vi "Random Competition.vi"() -> ()   [LabVIEW 2025]
uses:
  <vilib>/numeric/Random Number (Range) DBL.vi
panel:
  out "Iteration Count":i32
  out "Winner B":bool
  out "Tie":bool
  out "Winner A":bool
  out "Points B":dbl
  out "Points A":dbl
  out "Random Number B":dbl
  out "Random Number A":dbl
  in  "Number of Iterations":i32 min=0 step=1
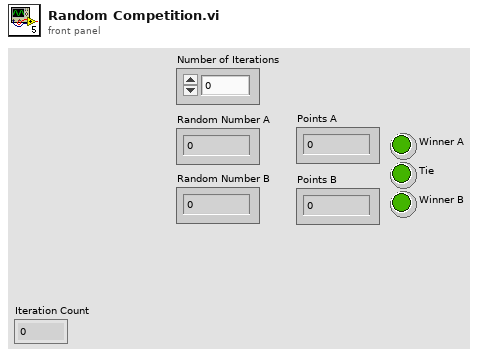
[diagram p1: front panel]
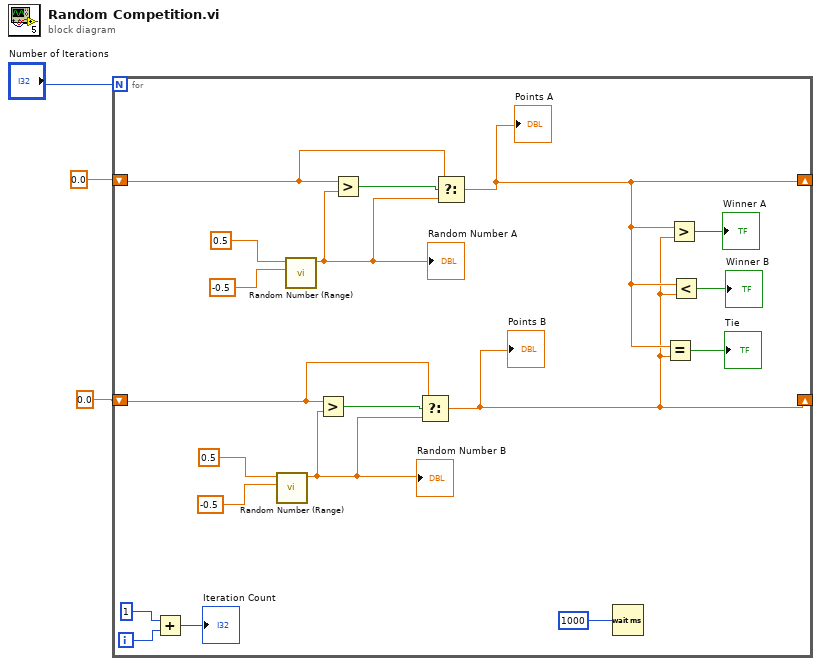
[diagram p0: block diagram]
diagram:
  n1 = for {
    N: "Number of Iterations" -> [_]
    shift-right: [w11] -> _
    shift-left: 0.0 -> [w17]
    shift-right: [w10] -> _
    shift-left: 0.0 -> [w12]
    i -> [w21]
    n2 = Add(x=1, y=w21) -> (x+y=→"Iteration Count":i32)
    n3 = call-poly <vilib>:"Random Number (Range).vi"("lower bound (0)"=-0.5, "upper bound (100)"=0.5) -> ("number"=w9:dbl)  [unwired: 9 in]
    "Random Number B" <- w9
    n4 = call-poly <vilib>:"Random Number (Range).vi"("lower bound (0)"=-0.5, "upper bound (100)"=0.5) -> ("number"=w8:dbl)  [unwired: 9 in]
    "Random Number A" <- w8
    n5 = Greater?(x=w12, y=w9) -> (0:w13:bool)
    n6 = Greater?(x=w17, y=w8) -> (0:w18:bool)
    n7 = Select(t=w12, s=w13, f=w9) -> (s? t:f=w10:dbl)
    "Points B" <- w10
    n8 = Select(t=w17, s=w18, f=w8) -> (s? t:f=w11:dbl)
    "Points A" <- w11
    n9 = Wait (ms)(milliseconds to wait=u32 1000) -> ()  [unwired: 1 out]
    n10 = Equal?(x=w11, y=w10) -> (x = y?=→"Tie":bool)
    n11 = Greater?(x=w11, y=w10) -> (0:→"Winner A":bool)
    n12 = Less?(x=w11, y=w10) -> (x < y?=→"Winner B":bool)
  }
